vi "signal_mutation.vi"(6 "scan points cluster in":T1, 7 "amplitude compensation?":bool, 8 "FPGA parameters in":T3 {"AOD center frequ. (Hz)_y" format="%.14g"; "AOD half bandwidth_y" format="%.14g"; "AOD Bandwidth_y (Hz)" format="%_6f"; "AOD center frequ. (Hz)_x" format="%.14g"; "cos Phi" format="%.35g"; "sin Phi" format="%.35g"; "AOD_Scale_Factor (1/Zoom)" format="%.35g"; "AOD half bandwidth_x" format="%.14g"; "AOD Bandwidth_x (Hz)" format="%_6f"}, 9 "acquire?":bool, 10 "y point bandwidth":fxp<+,36,32> format="%.28g", 11 "x point bandwidth":fxp<+,36,32> format="%.28g") -> (0 "FPGA parameters out":T3 {"AOD center frequ. (Hz)_y" format="%.14g"; "AOD half bandwidth_y" format="%.14g"; "AOD Bandwidth_y (Hz)" format="%_6f"; "AOD center frequ. (Hz)_x" format="%.14g"; "cos Phi" format="%.35g"; "sin Phi" format="%.35g"; "AOD_Scale_Factor (1/Zoom)" format="%.35g"; "AOD half bandwidth_x" format="%.14g"; "AOD Bandwidth_x (Hz)" format="%_6f"}, 3 "cluster out":T2)   [LabVIEW 2010]
uses:
  FPGA_parameters_cluster.ctl
  DDS_board_values_cluster.ctl
  scan_points_cluster.ctl
panel:
  in  "cluster constant":T2
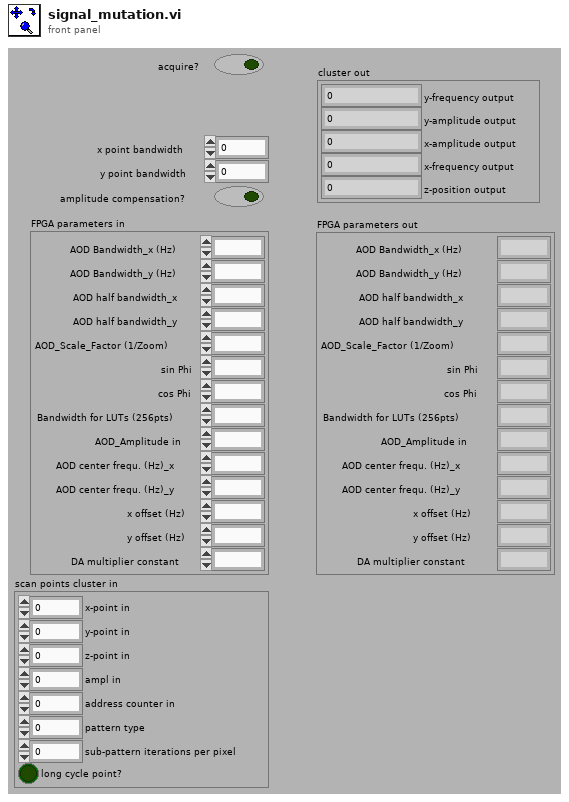
[diagram p1: front panel]
types:
  T1 = typedef "scan_points_cluster.ctl" = cluster{"x-point in":u16, "y-point in":u16, "z-point in":u16, "ampl in":u16, "address counter in":i32, "pattern type":i8, "sub-pattern iterations per pixel":u16, "long cycle point?":bool}
  T2 = typedef "DDS_board_values_cluster.ctl" = cluster{"y-frequency output":fxp<+,36,32>, "y-amplitude output":u16, "x-amplitude output":u16, "x-frequency output":fxp<+,36,32>, "z-position output":i16}
  T3 = typedef "FPGA_parameters_cluster.ctl" = cluster{"AOD Bandwidth_x (Hz)":fxp<+,36,32>, "AOD Bandwidth_y (Hz)":fxp<+,36,32>, "AOD half bandwidth_x":fxp<+,36,32>, "AOD half bandwidth_y":fxp<+,36,32>, "AOD_Scale_Factor (1/Zoom)":fxp<+,36,2>, "sin Phi":fxp<+/-,36,2>, "cos Phi":fxp<+/-,36,2>, "Bandwidth for LUTs (256pts)":fxp<+,36,0>, "AOD_Amplitude in":u16, "AOD center frequ. (Hz)_x":fxp<+,36,32>, "AOD center frequ. (Hz)_y":fxp<+,36,32>, "x offset (Hz)":fxp<+/-,36,32>, "y offset (Hz)":fxp<+/-,36,32>, "DA multiplier constant":fxp<+,64,4>}
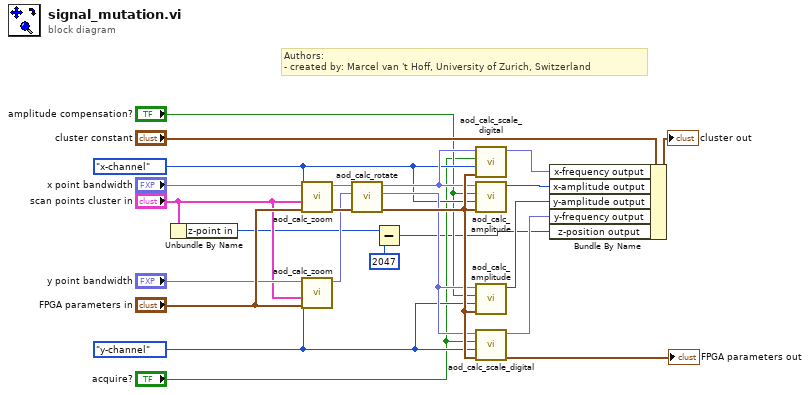
[diagram p0: block diagram]
diagram:
  w7 = enum16{"x-channel", "y-channel"}."y-channel" ("channel selector in")
  w8 = enum16{"x-channel", "y-channel"}."x-channel" ("channel selector in")
  # "Authors: \n- created by: Marcel van 't Hoff, University of Zurich, Switzerland"
  n1 = Unbundle By Name("scan points cluster in") -> ("z-point in"=w2:u16)
  n2 = call "aod_calc_zoom.vi"("FPGA parameters in"="FPGA parameters in", "scan points cluster in"="scan points cluster in", "channel selector in"=w8, "point bandwidth"="x point bandwidth") -> ("FPGA parameters out"=w22:T3, "scaled output"=w19:fxp<+/-,36,32>)  [unwired: 6 in]
  n3 = call "aod_calc_zoom.vi"("FPGA parameters in"="FPGA parameters in", "scan points cluster in"="scan points cluster in", "channel selector in"=w7, "point bandwidth"="y point bandwidth") -> ("scaled output"=w20:fxp<+/-,36,32>)  [unwired: 6 in, 1 out]
  n4 = call "aod_calc_rotate.vi"("FPGA parameters in"=w22, "scaled y input"=w20, "scaled x input"=w19) -> ("FPGA parameters out"=w23:T3, "y rotation out"=w16:fxp<+/-,36,32>, "x rotation out"=w15:fxp<+/-,36,32>)  [unwired: 6 in]
  n5 = Subtract(x=w2, y=u16 2047) -> (x-y=w1:i16)
  n6 = call "aod_calc_scale_digital.vi"("FPGA parameters in"=w23, "channel selector in"=w8, "acquire?"="acquire?", "input"=w15) -> ("output"=w13:fxp<+,36,32>)  [unwired: 6 in, 1 out]
  n7 = call "aod_calc_amplitude.vi"("FPGA parameters in"=w23, "channel selector in"=w8, "amplitude compensation?"="amplitude compensation?", "scaled input"=w15) -> ("output"=w12:u16)  [unwired: 6 in, 1 out]
  n8 = call "aod_calc_amplitude.vi"("FPGA parameters in"=w23, "channel selector in"=w7, "amplitude compensation?"="amplitude compensation?", "scaled input"=w16) -> ("output"=w11:u16)  [unwired: 6 in, 1 out]
  n9 = call "aod_calc_scale_digital.vi"("FPGA parameters in"=w23, "channel selector in"=w7, "acquire?"="acquire?", "input"=w16) -> ("FPGA parameters out"=→"FPGA parameters out":T3, "output"=w10:fxp<+,36,32>)  [unwired: 6 in]
  n10 = Bundle By Name(cluster="cluster constant", "x-frequency output"=w13, "x-amplitude output"=w12, "y-amplitude output"=w11, "y-frequency output"=w10, "z-position output"=w1) -> (→"cluster out":T2)
